vi "CreatePrivateEvents.vi"(8 "error in (no error)":errorcluster, 11 "Microscope":refnum<class "Microscope.lvclass">) -> (0 "error out":errorcluster, 3 "Microscope out":refnum<class "Microscope.lvclass">)   [LabVIEW 2013, in "Microscope.lvclass"]
doc: "JKI State Machine Objects (SMO) 1.0.2.13\nJKI - JKI\nCopyright (c) 2016, JKI"
uses:
  Microscope.lvclass
  <vilib>/JKI/JKI SMO/SMO/SMO.lvclass
  Typedefs/NewValueEvent--Cluster.ctl
  Typedefs/PrivateEvents--Microscope.Initialize.ctl
  Typedefs/PrivateEvents--Microscope.CaptureImageAtPosition.ctl
  XYStage/Typedefs/(real)Coords--Cluster.ctl
  XYStage/XYStage.lvclass
panel:
  # "For instructions on how to use the JKI State Machine Objects, examples and video tutorials, visit:\nhttp://jki.net/state-machine-objects/\n\nJKI State Machine Objects™\nhttp://jki.net/state-machine-objects/\nCopyright (C) 2005-2015, JKI <info@jki.net>\nALL RIGHTS RESERVED"
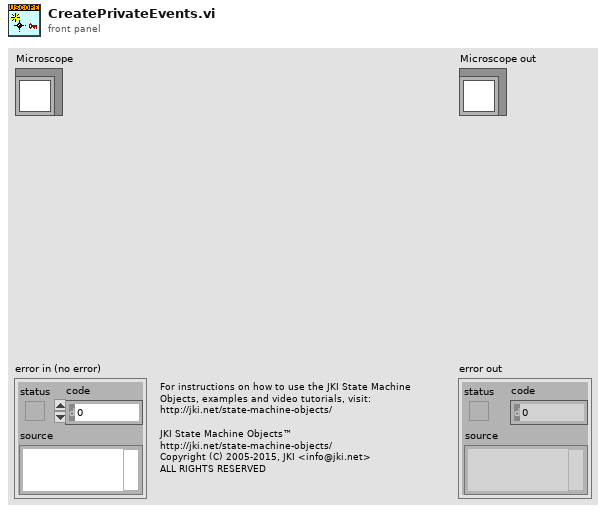
[diagram p1: front panel]
types:
  T1 = typedef "Microscope.lvclass/PrivateData--Ref.ctl" = refnum<data-value>
  T2 = typedef "Microscope.lvclass/PrivateEvents--Microscope.CaptureImageAtPosition.ctl" = cluster{"Coords":T3, "image notifier":refnum<notifier>, "Move?":bool}
  T3 = typedef "XYStage.lvclass/(real)Coords--Cluster.ctl" = cluster{"X":dbl, "Y":dbl}
  T4 = typedef "Microscope.lvclass/PrivateEvents--Microscope.Initialize.ctl" = bool
  T5 = typedef "Microscope.lvclass/NewValueEvent--Cluster.ctl" = cluster{"Value":string}
  T6 = typedef "Microscope.lvclass/PrivateData--Cluster.ctl" = cluster{"Public Events":T7, "Protected Events":T8, "Private Events":T9, "Dependencies":T10, "Configuration":T11}
  T7 = typedef "Microscope.lvclass/PublicEvents--Cluster.ctl" = cluster{"Value Changed":refnum<user-event>, "Initialized":refnum<user-event>}
  T8 = typedef "Microscope.lvclass/ProtectedEvents--Cluster.ctl" = cluster{"placeholder":refnum<user-event>}
  T9 = typedef "Microscope.lvclass/PrivateEvents--Cluster.ctl" = cluster{"New Value":refnum<user-event>, "Initialize":refnum<user-event>, "CaptureImageAtPosition":refnum<user-event>}
  T10 = typedef "Microscope.lvclass/Dependencies--Cluster.ctl" = cluster{"XYStage":refnum<class "XYStage.lvclass">, "Camera":refnum<class "Camera.lvclass">}
  T11 = typedef "Microscope.lvclass/Configuration--Cluster.ctl" = cluster{"XY Stage":string, "Camera":string, "image output folder":path, "filetype":string}
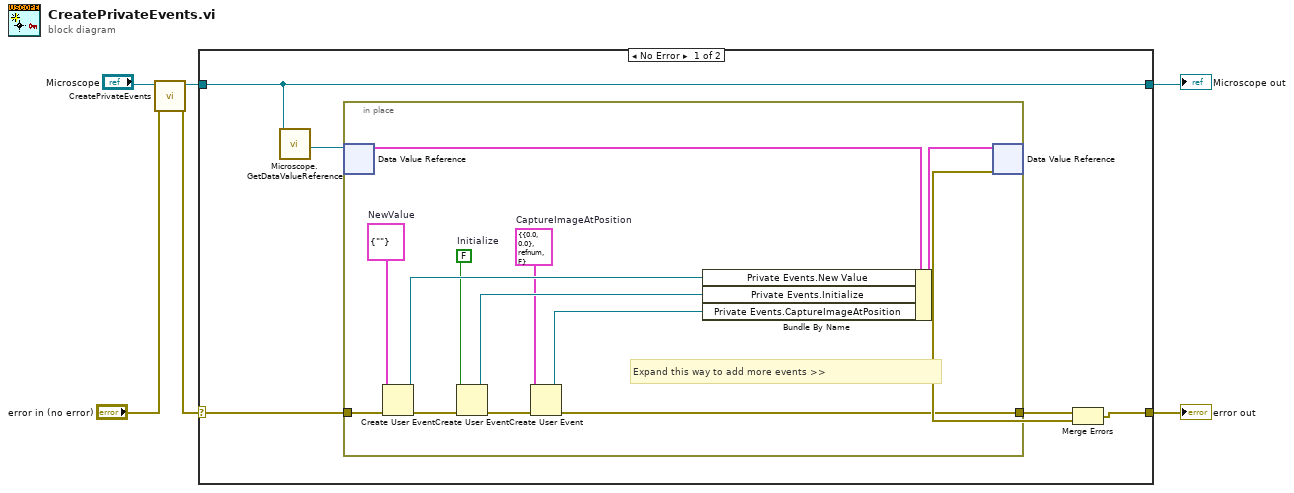
[diagram p0: block diagram]
diagram:
  n1 = call-parent "CreatePrivateEvents.vi"("error in (no error)"="error in (no error)", "SMO"="Microscope") -> ("error out"=w5:errorcluster, "SMO out"=w6:refnum<class "Microscope.lvclass">)  [unwired: 8 in]
  n2 = case shown="No Error" w5 {
    selector: w5 -> [w12 w26]
    tunnel: [w11 w26] -> w1
    tunnel: [w8 w25] -> w3
    tunnel: w6 -> [w8 w25]
    frame No Error {
      n3 = call "Microscope.GetDataValueReference.vi"("Microscope"=w8) -> ("Ref"=w7:T1)  [unwired: 10 in]
      n4 = in-place {
        in-place-border: w12 -> [w22]
        in-place-border: [w15] -> w10
        w14 = T2 {"Coords"={"X"=0.0, "Y"=0.0}, "image notifier"=refnum, "Move?"=FALSE}  # CaptureImageAtPosition
        w17 = T4 FALSE  # Initialize
        w19 = T5 {"Value"=""}  # NewValue
        # "Expand this way to add more events >>"
        n5 = in-place-dvr #1(w7) -> (w21:T6)  [unwired: 1 out]
        n6 = Create User Event(user event datatype=w19, error in=w22) -> (user event=w20:refnum<user-event>, error out=w23:errorcluster)
        n7 = Create User Event(user event datatype=w17, error in=w23) -> (user event=w16:refnum<user-event>, error out=w18:errorcluster)
        n8 = Create User Event(user event datatype=w14, error in=w18) -> (user event=w13:refnum<user-event>, error out=w15:errorcluster)
        n9 = Bundle By Name(cluster=w21, "Private Events.New Value"=w20, "Private Events.Initialize"=w16, "Private Events.CaptureImageAtPosition"=w13) -> (w24:T6)
        n10 = in-place-dvr #1(w24) -> (w9:errorcluster)  [unwired: 1 out]
      }
      n11 = Merge Errors(w10, w9) -> (w11:errorcluster)
    }
    frame Error {
    }
  }
  "error out" <- w1
  "Microscope out" <- w3
